vi "Calcolo NPSH3_.vi"(7 "% caduta":dbl=3.0 format="%#_13g", 8 "Cluster in":cluster{"index":i32, "length":i32}, 9 "Htot":dbl[](array[numeric]), 10 "Htot ref[m]":dbl[](array[numeric]), 11 "npsh":dbl[](array[numeric])) -> (0 "Graph interp":cluster{dbl[], dbl[]}, 1 "Graph":cluster{dbl[], dbl[]}, 2 "Htot-3%":dbl, 3 "Npsh3%":dbl)   [LabVIEW 2019]
uses:
  <vilib>/gmath/NI_Gmath.lvlib
panel:
  out "Htot ref":dbl
  out "XY Graph":cluster{dbl[], dbl[]}[](graph)
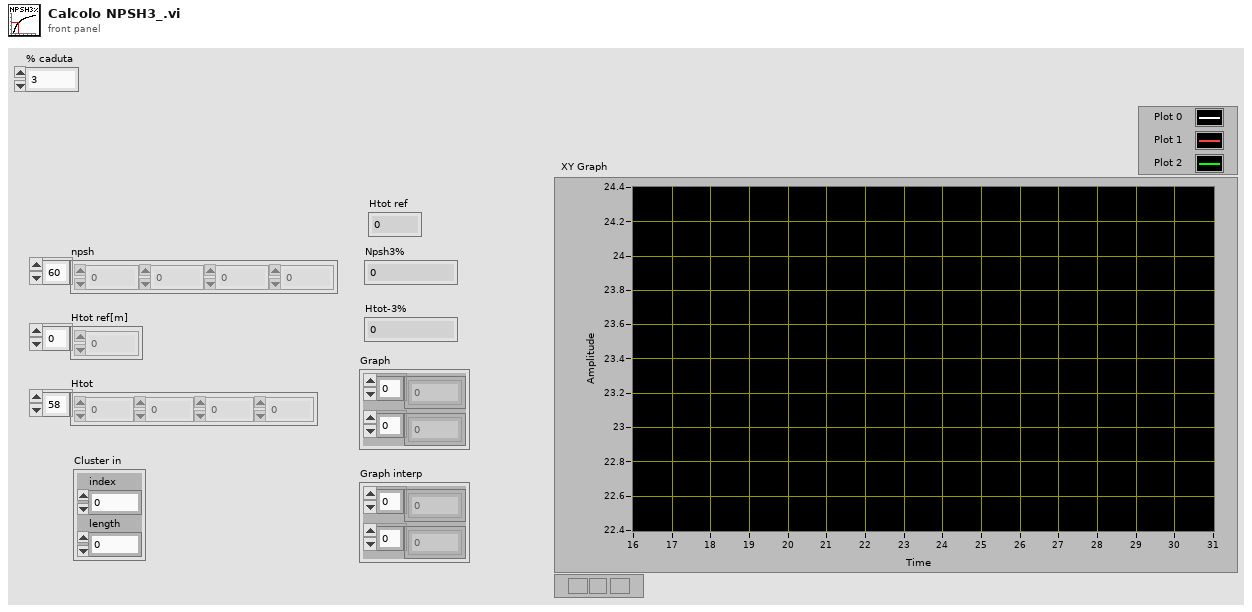
[diagram p1: front panel]
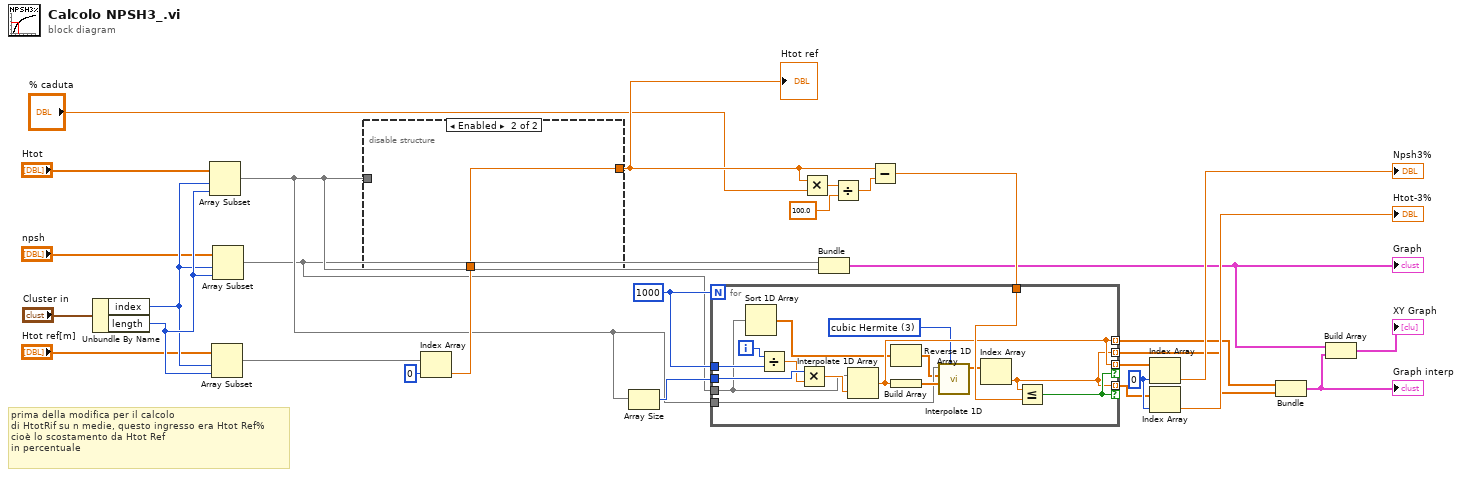
[diagram p0: block diagram]
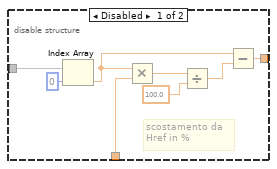
[diagram p2: hidden frame]
diagram:
  w23 = 0 ("index")
  w11 = 1000
  # "prima della modifica per il calcolo\ndi HtotRif su n medie, questo ingresso era Htot Ref%\ncioè lo scostamento da Htot Ref \nin percentuale"
  n1 = Unbundle By Name("Cluster in") -> ("index"=w14:i32, "length"=w15:i32)
  n2 = Array Subset(array="Htot", index=w14, length=w15) -> (w2:dbl[])
  n3 = Array Subset(array="Htot ref[m]", index=w14, length=w15) -> (w26:dbl[])
  n4 = Array Subset(array="npsh", index=w14, length=w15) -> (w1:dbl[])
  n5 = Index Array(array=w26, index=0) -> (element=w27:dbl)
  n6 = disable-structure shown="Enabled" {
    disable-tunnel: [w37 w38] -> w28
    disable-tunnel: w27 -> [w36 w38]
    disable-tunnel: w2 -> [w30 _]
    frame Disabled {
      # "scostamento da \nHref in %"
      n7 = Index Array(array=w30, index=0) -> (element=w35:dbl)
      n8 = Multiply(x=w35, y=w36) -> (x*y=w31:dbl)
      n9 = Divide(x=w31, y=100.0) -> (x/y=w33:dbl)
      n10 = Subtract(x=w35, y=w33) -> (x-y=w37:dbl)
    }
    frame Enabled {
    }
  }
  "Htot ref" <- w28
  n11 = Array Size(array=w2) -> (size(s)=w6:i32)
  n12 = Multiply(x=w28, y="% caduta") -> (x*y=w17:dbl)
  n13 = Bundle(w1, w2) -> (w10:cluster{dbl[], dbl[]})  [unwired: 1 in]
  "Graph" <- w10
  n14 = Divide(x=w17, y=100.0) -> (x/y=w19:dbl)
  n15 = Subtract(x=w28, y=w19) -> (x-y=w20:dbl)
  n16 = for {
    N: w11 -> [_]
    tunnel: w2 -> [w42]
    tunnel: w1 -> [w40]
    tunnel: w6 -> [w54]
    tunnel: w11 -> [w51]
    tunnel: [w45] -> w7 mode=indexing
    tunnel: [w47] -> w8 mode=indexing
    tunnel: w20 -> [w50]
    tunnel: [w45] -> w22 mode=indexing if=w49
    tunnel: [w47] -> w21 mode=indexing if=w49
    i -> [w53]
    w44 = 3 items=["nearest", "linear", "spline", "cubic Hermite", "Lagrange"] ("method")
    n17 = Sort 1D Array(array=w40) -> (sorted array=w41:dbl[])
    n18 = Divide(x=w53, y=w51) -> (x/y=w52:dbl)
    n19 = Multiply(x=w54, y=w52) -> (x*y=w48:dbl)
    n20 = Interpolate 1D Array(1:w48, 2:w40) -> (0:w47:dbl)
    n21 = Reverse 1D Array(array=w41) -> (reversed array=w39:dbl[])
    n22 = Build Array(w47) -> (w46:dbl[])
    n23 = call <vilib>:"Interpolate 1D.vi"("method"=w44, "xi"=w46, "X"=w39, "Y"=w42) -> ("yi"=w43:dbl[])  [unwired: 5 in, 2 out]
    n24 = Index Array(array=w43) -> (element=w45:dbl)  [unwired: 1 in]
    n25 = Less Or Equal?(x=w45, y=w50) -> (x <= y?=w49:bool)
  }
  n26 = Index Array(array=w21, index=w23) -> (element=→"Npsh3%":dbl)
  n27 = Index Array(array=w22, index=w23) -> (element=→"Htot-3%":dbl)
  n28 = Bundle(w8, w7) -> (w5:cluster{dbl[], dbl[]})  [unwired: 1 in]
  "Graph interp" <- w5
  n29 = Build Array(w10, w5) -> (→"XY Graph":cluster{dbl[], dbl[]}[])
